vi "FGV_N_actual.vi"(3 "error in (no error)":errorcluster, 4 "N_actual in":i32, 5 "action":enum16{"increment", "set_start", "get"}(ring)=enum."get") -> (0 "error out":errorcluster, 1 "N_actual out":i32)   [LabVIEW 2019, in "Prueba031.lvclass"]
uses:
  Prueba031.lvclass
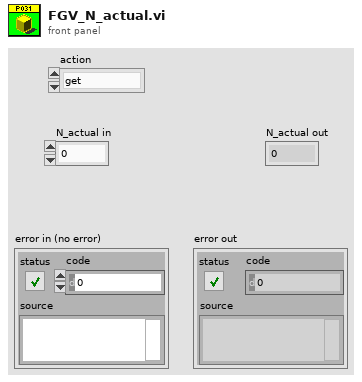
[diagram p1: front panel]
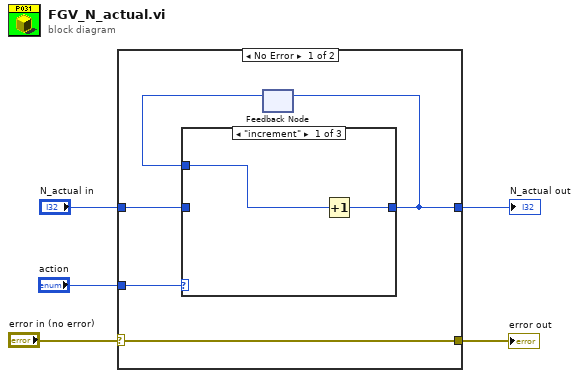
[diagram p0: block diagram]
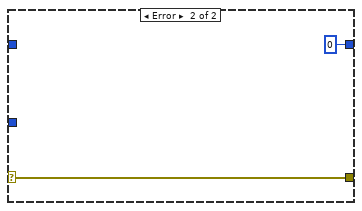
[diagram p4: hidden frame]
diagram:
  n1 = case shown="No Error" "error in (no error)" {
    selector: "error in (no error)" -> [w6 w16]
    tunnel: "action" -> [w10 _]
    tunnel: [w8 0 ("fila_inicial")] -> w4
    tunnel: "N_actual in" -> [w7 _]
    tunnel: [w6 w16] -> w1
    frame No Error {
      n2 = feedback #1() -> (w9:i32)  [unwired: 1 in]
      n3 = case shown="\"increment\"" w10 {
        tunnel: w9 -> [w11 w13 _]
        tunnel: [w12 w13 w14] -> w8
        tunnel: w7 -> [_ _ w14]
        frame "increment" {
          n4 = Increment(x=w11) -> (x+1=w12:i32)
        }
        frame "get", Default {
        }
        frame "set_start" {
        }
      }
      n5 = feedback-in #1(w8) -> ()
    }
    frame Error {
    }
  }
  "N_actual out" <- w4
  "error out" <- w1
